vi "Init Device.vi"(8 "error in (no error)":errorcluster, 10 "Settings":T1={"Simulation"=enum."off", "Exposure_Time"={"Value"=0.0, "Min"=0.0, "Max"=0.0, "StepSize"=0.0, "Tolerance"=0.0, "valueactual"=0.0}, "Timeout"={"Value"=0.0, "Min"=0.0, "Max"=0.0, "StepSize"=0.0, "Tolerance"=0.0, "valueactual"=0.0}, "External_Trigger"=enum."off", "Save"=enum."off", "CorrectSensitivity"=enum."off", "LocalSavingPath"=path "c:/temp"}, 11 "Qred in":refnum<class "Qred.lvclass">) -> (0 "error out":errorcluster, 2 "Device":string, 3 "Qred out":refnum<class "Qred.lvclass">)   [LabVIEW 2020, in "Qred.lvclass"]
uses:
  Qred.lvclass
  settingsQred_TypDef.ctl
  OnOffTypeDef.ctl
  C:/GEECS/Developers Version/builds/Device builds/Qred/RgbDriverKit.dll
  RgbDriverKit.dll
  Qred.lvclass/Qred.ctl
panel:
  out "Wavelengths":dbl[](array[numeric])
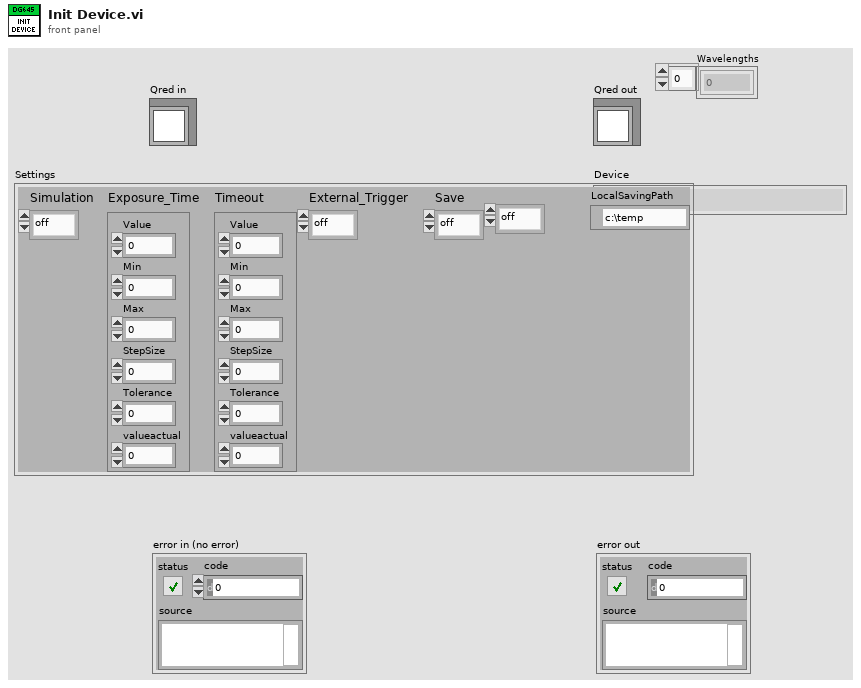
[diagram p1: front panel]
types:
  T1 = typedef "Qred.lvclass/settingsQred_TypDef.ctl" = cluster{"Simulation":T2, "Exposure_Time":cluster{"Value":dbl, "Min":dbl, "Max":dbl, "StepSize":dbl, "Tolerance":dbl, "valueactual":dbl}, "Timeout":cluster{"Value":dbl, "Min":dbl, "Max":dbl, "StepSize":dbl, "Tolerance":dbl, "valueactual":dbl}, "External_Trigger":T2, "Save":T2, "CorrectSensitivity":T2, "LocalSavingPath":path}
  T2 = typedef "OnOffTypeDef.ctl" = enum16{"off", "on"}
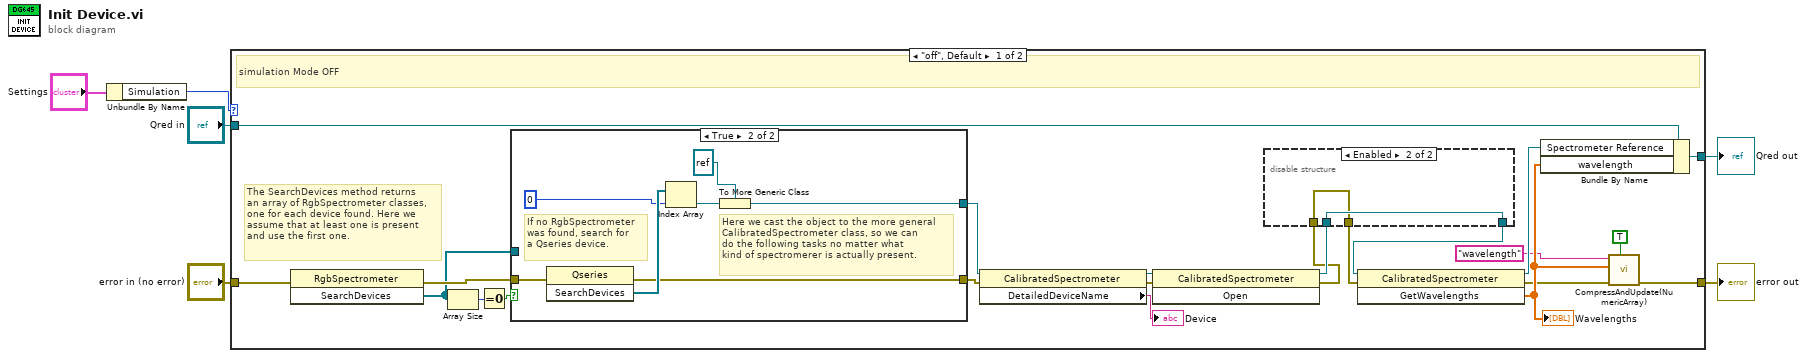
[diagram p0: block diagram]
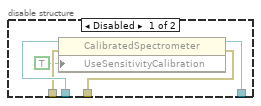
[diagram p2: hidden frame]
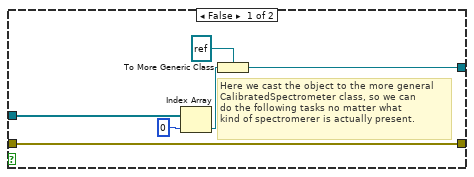
[diagram p3: hidden frame]
diagram:
  n1 = Unbundle By Name("Settings") -> ("Simulation"=w5:T2)
  n2 = case shown="\"off\", Default" w5 {
    tunnel: "error in (no error)" -> [w24 w49]
    tunnel: [w12 w49] -> w2
    tunnel: "Qred in" -> [w18 w50]
    tunnel: [w17 w50] -> w3
    frame "off", Default {
      # "The SearchDevices method returns\nan array of RgbSpectrometer classes,\none for each device found. Here we\nassume that at least one is present\nand use the first one."
      # "simulation Mode OFF"
      n3 = invoke class="RgbSpectrometer" method="SearchDevices"(error in=w24) -> (error out=w28:errorcluster, "SearchDevices"=w27:refnum<k24>[])  [unwired: 2 in, 1 out]
      n4 = Array Size(array=w27) -> (size(s)=w25:i32)
      n5 = Equal To 0?(x=w25) -> (x = 0?=w26:bool)
      n6 = case shown="True" w26 {
        tunnel: w28 -> [w38 w48]
        tunnel: w27 -> [w37 _]
        tunnel: [w36 w42] -> w20
        tunnel: [w38 w45] -> w19
        frame False {
          # "Here we cast the object to the more general\nCalibratedSpectrometer class, so we can\ndo the following tasks no matter what\nkind of spectromerer is actually present."
          n7 = Index Array(array=w37, index=0) -> (element=w40:refnum<k24>)
          n8 = To More Generic Class(target class=refnum<k24> refnum, reference=w40) -> (generic class reference=w36:refnum<k24>)
        }
        frame True {
          # "If no RgbSpectrometer\nwas found, search for\na Qseries device."
          # "Here we cast the object to the more general\nCalibratedSpectrometer class, so we can\ndo the following tasks no matter what\nkind of spectromerer is actually present."
          n9 = invoke class="Qseries" method="SearchDevices"(error in=w48) -> (error out=w45:errorcluster, "SearchDevices"=w47:refnum<k24>[])  [unwired: 2 in, 1 out]
          n10 = Index Array(array=w47, index=0) -> (element=w44:refnum<k24>)
          n11 = To More Generic Class(target class=refnum<k24> refnum, reference=w44) -> (generic class reference=w42:refnum<k24>)
        }
      }
      n12 = property class="CalibratedSpectrometer"(reference=w20, error in=w19) -> (reference out=w23:refnum<k24>, error out=w22:errorcluster, "DetailedDeviceName"=→"Device":string)
      n13 = invoke class="CalibratedSpectrometer" method="Open"(reference=w23, error in=w22) -> (reference out=w10:refnum<k24>, error out=w8:errorcluster)  [unwired: 1 in, 1 out]
      n14 = disable-structure shown="Enabled" {
        disable-tunnel: w10 -> [w33 w35]
        disable-tunnel: [w32 w35] -> w9
        disable-tunnel: w8 -> [w31 w34]
        disable-tunnel: [w30 w34] -> w7
        frame Disabled {
          n15 = property class="CalibratedSpectrometer"(reference=w33, error in=w31, "UseSensitivityCalibration"=TRUE) -> (reference out=w32:refnum<k24>, error out=w30:errorcluster)
        }
        frame Enabled {
        }
      }
      n16 = invoke class="CalibratedSpectrometer" method="GetWavelengths"(reference=w9, error in=w7) -> (reference out=w16:refnum<k24>, error out=w13:errorcluster, "GetWavelengths"=w15:dbl[])  [unwired: 1 in]
      "Wavelengths" <- w15
      n17 = Bundle By Name(cluster=w18, "Spectrometer Reference"=w16, "wavelength"=w15) -> (w17:refnum<class "Qred.lvclass">)
      n18 = call "CompressAndUpdate(NumericArray).vi"("force CVT update (false)"=TRUE, "error in"=w13, "Numeric Array"=w15, "command or variable name"="wavelength") -> ("error out"=w12:errorcluster)  [unwired: 7 in]
    }
    frame "on" {
      # "Simulation Mode ON"
    }
  }
  "Qred out" <- w3
  "error out" <- w2
